vi "tb_interpolation_fft_simio_fpga.vi"() -> ()   [LabVIEW 2011]
uses:
  <vilib>/Platform/TimedLoop/XDataNode/XDataNode.xnode
  <vilib>/Platform/TimedLoop/XDataNode/nitl_modes.ctl
  <vilib>/Platform/TimedLoop/XDataNode/XDNodeRunTimeDep.lvlib
  <vilib>/Platform/TimedLoop/XDataNode/wakeup.ctl
  <vilib>/Platform/TimedLoop/XDataNode/timing_clust.ctl
  <vilib>/rvi/DataTransferAndStorage/Container/XNode/niFpgaContainer.xnode
  <vilib>/rvi/FXPMathLib/FxpInterpret/XNode/nifxpmath_Interpret.xnode
  <vilib>/eio/EIONode/EIONode.xnode
  <userlib>/FPGA Library/Code Development/Signal Processing/Interpolation Block/Controls/Interpolation Input Data.ctl
  <vilib>/rvi/FIFO/Fifo_Resource/nirvififoEmulationRead.vi
  <vilib>/rvi/FIFO/Fifo_Resource/nirvififoEmulationWrite.vi
  <vilib>/rvi/FIFO/Fifo_Resource/nirvififoEmulationGetNumberOfElementsToRead.vi
  <vilib>/rvi/interface/RandomDataEmulation/nirviRandomDataFpgaReadWriteTemplate.vi
  <vilib>/rvi/eio/common/nirviEmuTemplateMethod_errors.vi
  <userlib>/FPGA Library/Code Development/Signal Processing/FFT Block/FFT/Controls/FFT States.ctl
  <userlib>/FPGA Library/Code Development/Signal Processing/FFT Block/FFT/Controls/FFT Parameters.ctl
panel:
  out "ReFFT1":i16[](array[numeric])
  out "Real{FFT1}":i16(graph)
  out "Input Data":i16(graph)
  out "Interp Loop Overflow":bool
  out "Resampled Waveform":i16(graph)
  out "Current FFT State":T1
  out "FFT Input Valids":u64
  out "FFT Output Valids":u64
  out "FFT Status":T2
  in  "Address":u32
  in  "Data":T3 {"x[n].ResampleInfo"."Lambda" format="%.18g"; "x[n-1].ResampleInfo"."Lambda" format="%.18g"}
  in  "Write?":bool
  in  "FFT Parameters":T4={"Direction"=TRUE, "scale_sch"=85.0, "Flush Length"=0} {"scale_sch" format="%.0b"}
  in  "FFT State":cluster{"FFT State":T1, "Set FFT State?":bool}
  out "acq timed out?":bool
  out "Numeric":i32
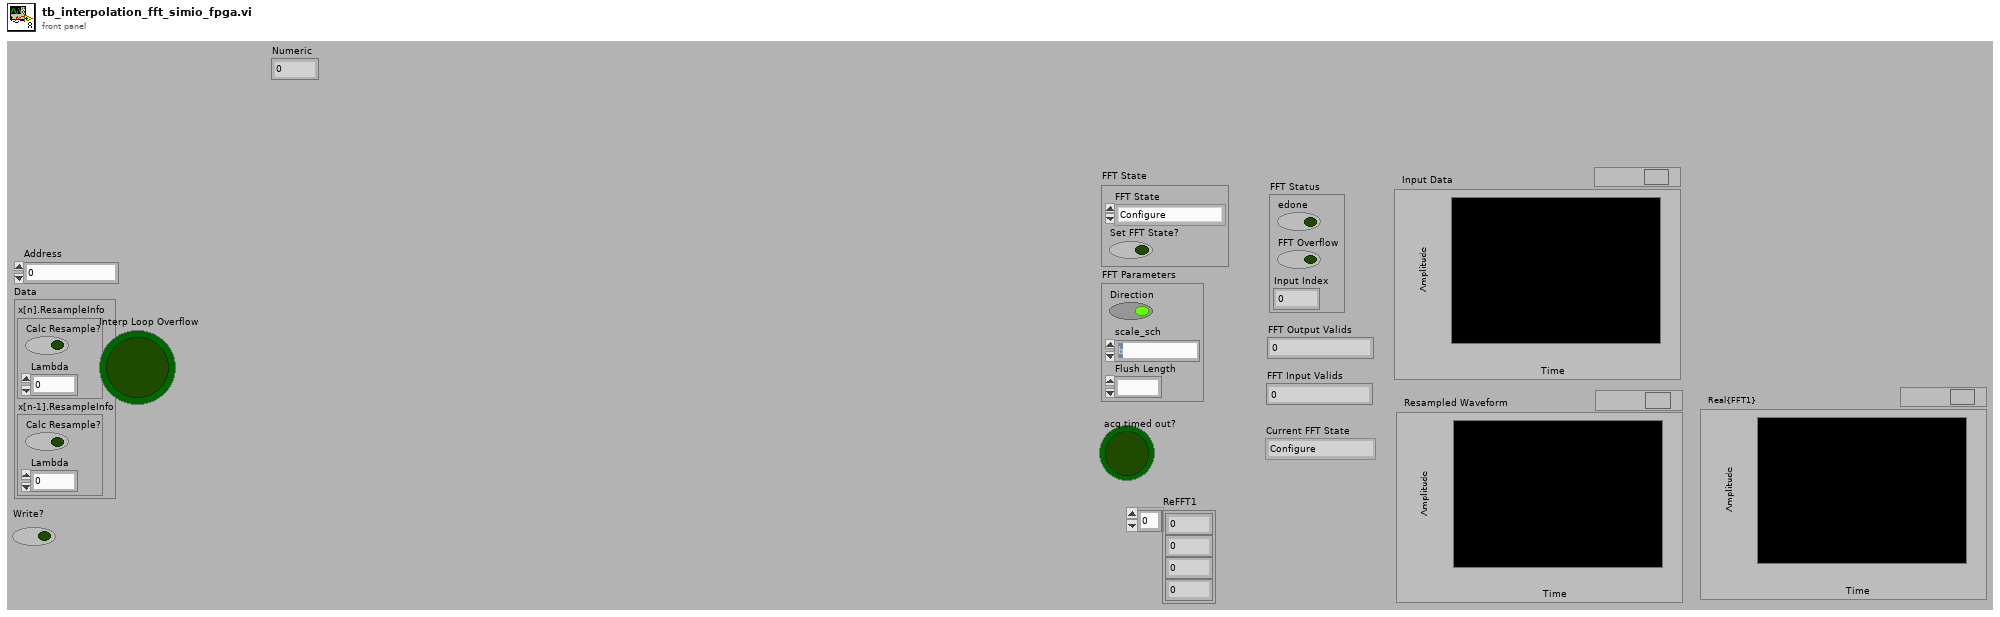
[diagram p1: front panel]
types:
  T1 = typedef "FFT States.ctl" = enum8{"Configure", "Start FFT processing", "Process", "Unload Last FFT", "Reset"}
  T2 = cluster{"edone":bool, "FFT Overflow":bool, "Input Index":fxp<+,9,9>}
  T3 = cluster{"x[n].ResampleInfo":cluster{"Calc Resample?":bool, "Lambda":fxp<+/-,18,1>}, "x[n-1].ResampleInfo":cluster{"Calc Resample?":bool, "Lambda":fxp<+/-,18,1>}}
  T4 = typedef "FFT Parameters.ctl" = cluster{"Direction":bool, "scale_sch":fxp<+,10,10>, "Flush Length":u16}
  T5 = typedef "XDNodeRunTimeDep.lvlib/timing_clust.ctl" = cluster{"Expected End [f-1]":u64, "Actual End [f-1]":u64, "Finished Late? [f-1]":bool, "Expected End [i-1]":u64, "Actual End [i-1]":u64, "Finished Late? [i-1]":bool, "Expected Start [i]":u64, "Actual Start [i]":u64, "Expected Start [f]":u64, "Actual Start [f]":u64, "Source Name":string, "Structure Name":string, "Period":i64, "Deadline":i64, "Offset":i64, "Start":i64, "Priority":i32, "Timeout":i32, "Mode":T6, "Wakeup Reason":T7, "Error":errorcluster, "Source Type":string, "Secondary Source Type":string, "Global End Time":u64, "Global Start Time":u64, "Frame Duration":u64, "Iteration Duration":u64, "Assigned CPU":i32, "I/O Scan Engine Mode":u32}
  T6 = typedef "XDNodeRunTimeDep.lvlib/nitl_modes.ctl" = enum32{"No Change", "Process missed periods, maintain original phase", "Discard missed periods, maintain original phase", "Process missed periods, ignore original phase", "Discard missed periods, ignore original phase"}
  T7 = typedef "XDNodeRunTimeDep.lvlib/wakeup.ctl" = enum32{"Normal", "Aborted", "Asynchronous wakeup", "Timing source error", "Timed loop error", "Timeout"}
  T8 = typedef "Interpolation Input Data.ctl" = fxp<+/-,18,1>
  T9 = typedef "Interpolation Output Data.ctl" = fxp<+/-,19,1>
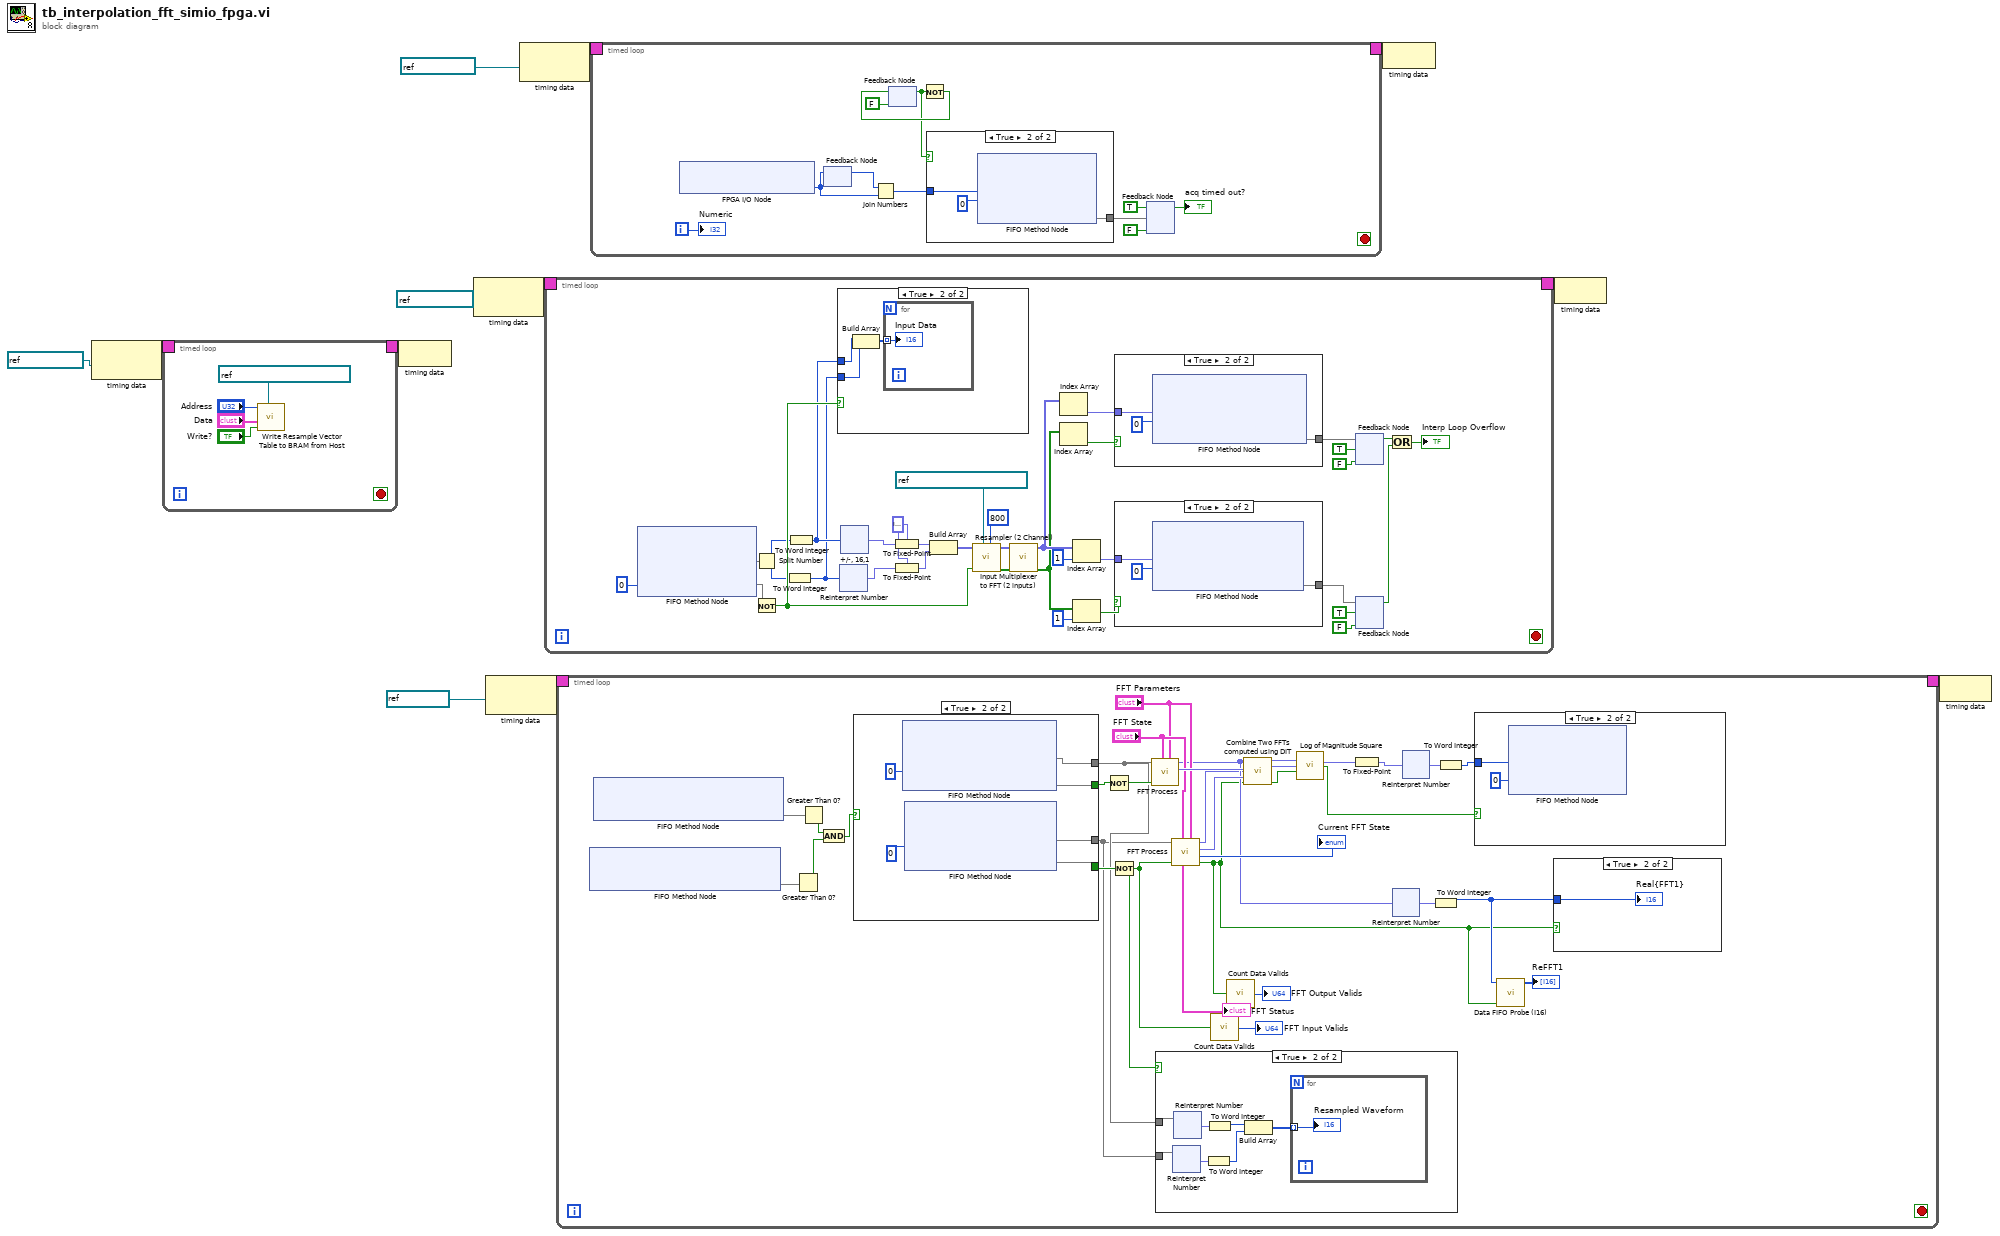
[diagram p0: block diagram]
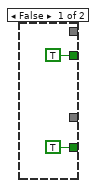
[diagram p9: hidden frame]
diagram:
  (unwired) refnum<k21> "126.67MHz" ("Source Name")
  n1 = node-c288(refnum<k21> "126.67MHz" ("Source Name")) -> (w5:T5)
  n2 = timed-loop {
    timing: w5 -> [_]
    timing-out: [_] -> w4
    stop <- _ stop-if-true
    n3 = call <userlib>:"Write Resample Vector Table to BRAM from Host.vi"("Resample Table"=refnum<k21> "Resample Vector Table", "Write?"="Write?", "Data"="Data", "Address"="Address") -> ()  [unwired: 8 in]
  }
  n4 = node-c288(w4) -> ()
  n5 = node-c288() -> (w2:T5)  [unwired: 1 in]
  n6 = node-c288(refnum<k21> "176MHz" ("Source Name")) -> (w11:T5)
  n7 = node-c288(refnum<k21> "ADC Clock" ("Source Name")) -> (w9:T5)
  n8 = timed-loop {
    timing: w2 -> [_]
    timing-out: [_] -> w1
    stop <- _ stop-if-true
    w30 = T8 0.0 ("Interpolate.Input Data")
    n9 = xnode ("FIFO Method Node")("Timeout"=0) -> ("Element"=w33, "Timed Out?"=w28)  [unwired: 1 in, 1 out]
    n10 = Not(x=w28) -> (.not. x?=w22:bool)
    n11 = Split Number(x=w33) -> (hi(x)=w21:u16, lo(x)=w20:u16)
    n12 = To Word Integer(number=w20) -> (16bit integer=w18:i16)
    n13 = To Word Integer(number=w21) -> (16bit integer=w19:i16)
    n14 = case shown="True" w22 {
      tunnel: w19 -> [_ w55]
      tunnel: w18 -> [_ w53]
      frame False {
      }
      frame True {
        n15 = Build Array(w55, w53) -> (w54:i16[])
        n16 = for {
          tunnel: w54 -> [w56] mode=indexing
          "Input Data" <- w56
        }
      }
    }
    n17 = xnode "Reinterpret Number"("x"=w18) -> ("y"=w26:fxp<+/-,16,1>)
    n18 = xnode "+/-, 16,1"("x"=w19) -> ("y"=w24:fxp<+/-,16,1>)
    n19 = To Fixed-Point(fixed-point type=w30, number=w24) -> (fixed-point=w25:T8)
    n20 = To Fixed-Point(fixed-point type=w30, number=w26) -> (fixed-point=w31:T8)
    n21 = Build Array(w25, w31) -> (w29:T8[])
    n22 = call <userlib>:"Resampler (2 Channel).vi"("CalibrationTable Length-1"=u16 800, "ResampleVectorInfo"=refnum<k21> "Resample Vector Table", "DataValid"=w22, "Input Data"=w29) -> ("Data Valid"=w51:bool[], "Interpolated Data"=w52:T9[])  [unwired: 6 in]
    n23 = call <userlib>:"Input Multiplexer to FFT (2 inputs).vi"("Input Data Valid Array"=w51, "Input Data"=w52) -> ("Output Data Valid Array"=w46:bool[], "Interchanged Data"=w48:T9[])  [unwired: 8 in]
    n24 = Index Array(array=w48) -> (element=w50:T9)  [unwired: 1 in]
    n25 = Index Array(array=w46) -> (element=w49:bool)  [unwired: 1 in]
    n26 = Index Array(array=w48, index=1) -> (element=w47:T9)
    n27 = Index Array(array=w46, index=1) -> (element=w45:bool)
    n28 = case shown="True" w49 {
      tunnel: w50 -> [_ w66]
      tunnel: [_ w64] -> w42
      frame False {
      }
      frame True {
        n29 = xnode ("FIFO Method Node")("Element"=w66, "Timeout"=0) -> ("Timed Out?"=w64)  [unwired: 1 in, 1 out]
      }
    }
    n30 = case shown="True" w45 {
      tunnel: w47 -> [_ w63]
      tunnel: [_ w61] -> w39
      frame False {
      }
      frame True {
        n31 = xnode ("FIFO Method Node")("Element"=w63, "Timeout"=0) -> ("Timed Out?"=w61)  [unwired: 1 in, 1 out]
      }
    }
    n32 = feedback-in #1(w42, TRUE) -> ()
    n33 = feedback #1(FALSE ("Timed Out?")) -> (w38:bool)
    n34 = feedback #2(FALSE ("Timed Out?")) -> (w35:bool)
    n35 = feedback-in #2(w39, TRUE) -> ()
    n36 = Or(x=w38, y=w35) -> (x .or. y?=→"Interp Loop Overflow":bool)
  }
  n37 = timed-loop {
    timing: w11 -> [_]
    timing-out: [_] -> w10
    stop <- _ stop-if-true
    n38 = xnode ("FIFO Method Node")() -> ("Number of Elements to Read"=w96)  [unwired: 1 in, 1 out]
    n39 = xnode ("FIFO Method Node")() -> ("Number of Elements to Read"=w97)  [unwired: 1 in, 1 out]
    n40 = Greater Than 0?(x=w96) -> (x > 0?=w94:bool)
    n41 = Greater Than 0?(x=w97) -> (x > 0?=w95:bool)
    n42 = And(x=w95, y=w94) -> (x .and. y?=w93:bool)
    n43 = case shown="True" w93 {
      tunnel: [TRUE ("Timed Out?") w133] -> w101
      tunnel: [_ w132] -> w80
      tunnel: [_ w131] -> w79
      tunnel: [TRUE ("Timed Out?") w130] -> w100
      frame False {
      }
      frame True {
        n44 = xnode ("FIFO Method Node")("Timeout"=0) -> ("Element"=w132, "Timed Out?"=w133)  [unwired: 1 in, 1 out]
        n45 = xnode ("FIFO Method Node")("Timeout"=0) -> ("Element"=w131, "Timed Out?"=w130)  [unwired: 1 in, 1 out]
      }
    }
    n46 = Not(x=w101) -> (.not. x?=w98:bool)
    n47 = Not(x=w100) -> (.not. x?=w76:bool)
    n48 = call <userlib>:"FFT Process.vi"("FFT Parameters"="FFT Parameters", "FFT State"="FFT State", "Input Valid"=w98, "Real Data In"=w80) -> ("Imag Data Out"=w90:fxp<+/-,16,1>, "Real Data Out"=w74:fxp<+/-,16,1>)  [unwired: 2 in, 4 out]
    n49 = case shown="True" w76 {
      tunnel: w80 -> [_ w114]
      tunnel: w79 -> [_ w113]
      frame False {
      }
      frame True {
        n50 = xnode "Reinterpret Number"("x"=w113) -> ("y"=w111:fxp<+/-,16,16>)
        n51 = xnode "Reinterpret Number"("x"=w114) -> ("y"=w112:fxp<+/-,16,16>)
        n52 = To Word Integer(number=w111) -> (16bit integer=w109:i16)
        n53 = To Word Integer(number=w112) -> (16bit integer=w110:i16)
        n54 = Build Array(w110, w109) -> (w108:i16[])
        n55 = for {
          tunnel: w108 -> [w115] mode=indexing
          "Resampled Waveform" <- w115
        }
      }
    }
    n56 = call <userlib>:"FFT Process.vi"("FFT Parameters"="FFT Parameters", "FFT State"="FFT State", "Input Valid"=w76, "Real Data In"=w79) -> ("Output Valid"=w69:bool, "Current FFT State"=→"Current FFT State":T1, "Imag Data Out"=w89:fxp<+/-,16,1>, "Real Data Out"=w73:fxp<+/-,16,1>, "FFT Status"=→"FFT Status":T2)  [unwired: 2 in, 1 out]
    n57 = call <userlib>:"Count Data Valids.vi"("Data Valid"=w76) -> ("Counter"=→"FFT Input Valids":u64)  [unwired: 14 in]
    n58 = call <userlib>:"Count Data Valids.vi"("Data Valid"=w69) -> ("Counter"=→"FFT Output Valids":u64)  [unwired: 14 in]
    n59 = call <userlib>:"Combine Two FFTs computed using DIT.vi"("Real FFT 1"=w74, "Imag FFT 1"=w90, "Real FFT 2"=w73, "Imag FFT 2"=w89, "Input Data Valid"=w69) -> ("Real FFT k"=w78:fxp<+/-,24,3>, "Imag FFT k"=w77:fxp<+/-,24,3>, "Output Valid"=w75:bool)  [unwired: 6 in, 2 out]
    n60 = call <userlib>:"Log of Magnitude Square.vi"("Real"=w78, "Imaginary"=w77, "Input Valid"=w75) -> ("Log Magnitude"=w82:fxp<+/-,34,12>, "Output Valid"=w91:bool)  [unwired: 11 in]
    n61 = To Fixed-Point(number=w82) -> (fixed-point=w81:fxp<+/-,16,8>)  [unwired: 1 in]
    n62 = xnode "Reinterpret Number"("x"=w74) -> ("y"=w71:fxp<+/-,16,16>)
    n63 = xnode "Reinterpret Number"("x"=w81) -> ("y"=w99:fxp<+/-,16,16>)
    n64 = To Word Integer(number=w71) -> (16bit integer=w70:i16)
    n65 = To Word Integer(number=w99) -> (16bit integer=w92:i16)
    n66 = case shown="True" w91 {
      tunnel: w92 -> [_ w127]
      frame False {
      }
      frame True {
        n67 = xnode ("FIFO Method Node")("Element"=w127, "Timeout"=0) -> ()  [unwired: 1 in, 2 out]
      }
    }
    n68 = call <userlib>:"Data FIFO Probe (I16).vi"("Valid"=w69, "Data"=w70) -> ("Array"=→"ReFFT1":i16[])  [unwired: 9 in]
    n69 = case shown="True" w69 {
      tunnel: w70 -> [_ w102]
      frame False {
      }
      frame True {
        "Real{FFT1}" <- w102
      }
    }
  }
  n70 = timed-loop {
    timing: w9 -> [_]
    timing-out: [_] -> w8
    i -> [w147]
    stop <- _ stop-if-true
    n71 = xnode "FPGA I/O Node"() -> ("IO Module\\AI 0 Data"=w143:i16)  [unwired: 1 in, 1 out]
    n72 = feedback-in #3(w143) -> ()
    n73 = feedback #3() -> (w144:i16)  [unwired: 1 in]
    n74 = Join Numbers(hi=w144, lo=w143) -> ((hi.lo)=w145:u32)
    n75 = feedback #4(FALSE) -> (w146:bool)
    n76 = Not(x=w146) -> (.not. x?=w153:bool)
    n77 = feedback-in #4(w153) -> ()
    n78 = case shown="True" w146 {
      tunnel: w145 -> [_ w156]
      tunnel: [_ w154] -> w150
      frame False {
      }
      frame True {
        n79 = xnode ("FIFO Method Node")("Element"=w156, "Timeout"=0) -> ("Timed Out?"=w154)  [unwired: 1 in, 1 out]
      }
    }
    n80 = feedback-in #5(TRUE, w150) -> ()
    n81 = feedback #5(FALSE) -> (→"acq timed out?":bool)
    "Numeric" <- w147
  }
  n82 = node-c288(w8) -> ()
  n83 = node-c288(w1) -> ()
  n84 = node-c288(w10) -> ()
